vi "SwitchBetweenStates.vi"(8 "spitCube":bool, 9 "feedCube":bool, 10 "lowerArm":bool, 11 "raiseArm":bool) -> (3 "Output State":T1)   [LabVIEW 2017]
uses:
  StatesTypeDef.ctl
panel:
  # "input to the VI"
  # "output from the VI"
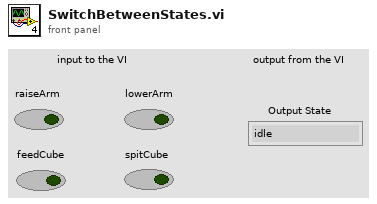
[diagram p1: front panel]
types:
  T1 = typedef "StatesTypeDef.ctl" = enum16{"idle", "lower", "raise", "feed", "spit"}
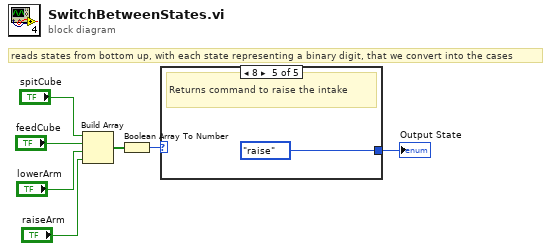
[diagram p0: block diagram]
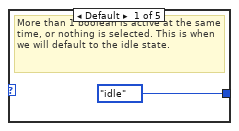
[diagram p2: hidden frame]
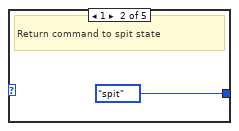
[diagram p3: hidden frame]
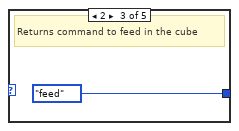
[diagram p4: hidden frame]
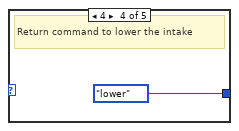
[diagram p5: hidden frame]
diagram:
  # "reads states from bottom up, with each state representing a binary digit, that we convert into the cases"
  n1 = Build Array("spitCube", "feedCube", "lowerArm", "raiseArm") -> (w5:bool[])
  n2 = Boolean Array To Number(Boolean array=w5) -> (number=w6:u32)
  n3 = case shown="8" w6 {
    tunnel: [StatesTypeDef."idle" ("Output State") StatesTypeDef."spit" ("Output State") StatesTypeDef."feed" ("Output State") StatesTypeDef."lower" ("Output State") StatesTypeDef."raise" ("Output State")] -> w7
    frame Default {
      # "More than 1 boolean is active at the same time, or nothing is selected. This is when we will default to the idle state."
    }
    frame 1 {
      # "Return command to spit state"
    }
    frame 2 {
      # "Returns command to feed in the cube"
    }
    frame 4 {
      # "Return command to lower the intake"
    }
    frame 8 {
      # "Returns command to raise the intake"
    }
  }
  "Output State" <- w7
